vi "Main.vi"(7 "Actor":refnum<class "Actor.lvclass">) -> ()   [LabVIEW 2020, in "_Template.lvlib" / "{{Actor}}.lvlib" / "Actor.lvclass"]
uses:
  Actor.lvclass
  Actor.lvclass/Actor.ctl
  C:/Users/nathan.davis/Desktop/personal/jettl-harness/repos/jettl/src/jettl Tools/_Template/{{Actor}}/ConcreteActor/Actor.lvclass
  C:/Users/nathan.davis/Desktop/personal/jettl-harness/repos/jettl/src/jettl Tools/_Template/{{Msg}}/ActorMessage/ActorMessage.lvclass
  C:/Users/nathan.davis/Desktop/personal/jettl-harness/repos/jettl/src/jettl/jettl/Actor/Actor.lvclass
  jettl/jettl/jettl.lvlib
types:
  T1 = cluster{"EventRegRef":refnum<event-registration>}
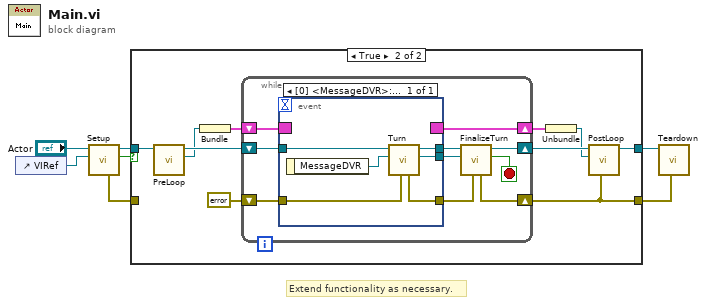
[diagram p0: block diagram]
diagram:
  # "Extend functionality as necessary."
  n1 = control-ref of="VIRef"() -> (w2:refnum<vi>)
  n2 = call "Setup.vi"("VIRef"=w2, "Actor"="Actor") -> ("BeginLoop"=w1:bool, "Actor"=w7:refnum<class "Actor.lvclass">, "Error"=w6:errorcluster)  [unwired: 7 in]
  n3 = case shown="True" w1 {
    tunnel: [w9 w14] -> w5
    tunnel: w7 -> [w9 w17]
    tunnel: [w8 w13] -> w4
    tunnel: w6 -> [w8 _]
    frame False {
    }
    frame True {
      n4 = call "PreLoop.vi"("Actor"=w17) -> ("EventRegRef"=w11:refnum<event-registration>, "Actor"=w16:refnum<class "Actor.lvclass">)  [unwired: 9 in]
      n5 = Bundle("EventRegRef"=w11) -> (w19:T1)  [unwired: 1 in]
      n6 = while {
        shift-right: [w23] -> w15
        shift-left: w16 -> [w29]
        shift-right: [w21] -> w18
        shift-left: w19 -> [w22]
        shift-right: [w26] -> w13
        shift-left: errorcluster {"status"=FALSE, "code"=0, "source"=""} ("Error") -> [w20]
        stop <- w28 stop-if-true
        n7 = event shown="[0] <MessageDVR>: User Event" {
          selector: w22 -> [_]
          dyn-events: [_] -> w21
          timeout: _ -> [_]
          tunnel: w29 -> [w35]
          tunnel: [w34] -> w24
          tunnel: [w33] -> w27
          tunnel: [w31] -> w25
          tunnel: w20 -> [w32]
          event User Event {
            n8 = event-data() -> ("MessageDVR"=w30:refnum<data-value>)  [unwired: 1 in]
            n9 = call "Turn.vi"("Error"=w32, "MessageDVR"=w30, "Actor"=w35) -> ("Message"=w31:refnum<class "Message.lvclass">, "Actor"=w34:refnum<class "Actor.lvclass">, "Error"=w33:errorcluster)  [unwired: 6 in]
          }
        }
        n10 = call "FinalizeTurn.vi"("Error"=w27, "Message"=w25, "Actor"=w24) -> ("Teardown"=w28:bool, "Actor"=w23:refnum<class "Actor.lvclass">, "Error"=w26:errorcluster)  [unwired: 6 in]
      }
      n11 = Unbundle(w18) -> ("EventRegRef"=w10:refnum<event-registration>)
      n12 = call "PostLoop.vi"("Error"=w13, "EventRegRef"=w10, "Actor"=w15) -> ("Actor"=w14:refnum<class "Actor.lvclass">)  [unwired: 8 in]
    }
  }
  n13 = call "Teardown.vi"("Error"=w4, "Actor"=w5) -> ()  [unwired: 9 in, 1 out]
